vi "FillSurfaceRects.vi"(8 "No Error":errorcluster, 9 "Color":u32, 10 "Rects":T1[](array[typedef]), 11 "Dst [SDL_Surface *]":i64 format="%.0x") -> (0 "error out":errorcluster)   [LabVIEW 2026, in "SDL3.lvlib" / "Surface.lvlib"]
doc: "<B>Summary</B>\nPerform a fast fill of a set of rectangles with a specific color.\n\n<B>Remarks</B>\ncolor should be a pixel of the format used by the surface, and can be generated by SDL_MapRGB() or SDL_MapRGBA(). If the color value contains an alpha component then the destination is simply filled with that alpha information, no blending takes place.\n\nIf there is a clip rectangle set on the destination (set via SDL_SetSurfaceClipRect()), then this function will fill based on the intersection of the clip rectangle and rect."
uses:
  Surface.lvlib
  Rect/Rect--cluster.ctl
  <vilib>/Utility/error.llb/Error Cluster From Error Code.vi
  Error/Error.lvlib
  Lib/SDL3.dll
  Rect/Rect.lvlib
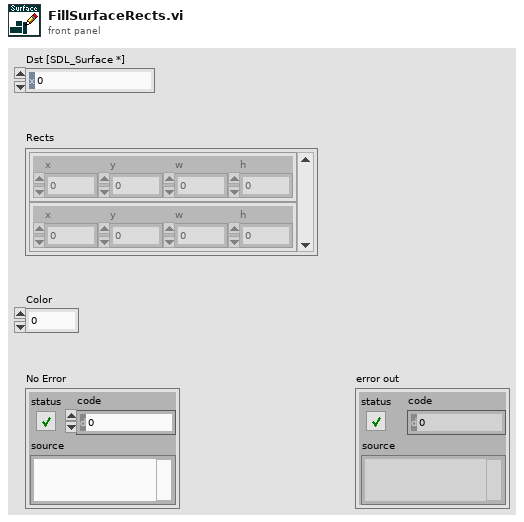
[diagram p1: front panel]
types:
  T1 = typedef "SDL3.lvlib/Rect.lvlib/Rect--cluster.ctl" = cluster{"x":i32, "y":i32, "w":i32, "h":i32}
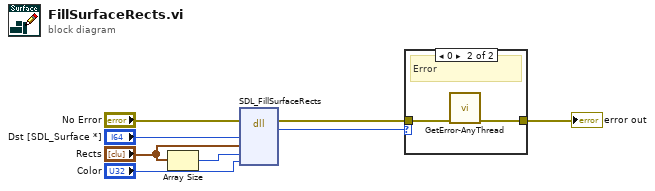
[diagram p0: block diagram]
diagram:
  n1 = Array Size(array="Rects") -> (size(s)=w1:i32)
  n2 = dll-call lib="C:/Users/saukko/Dev/LV-SDL3/Sources/SDL3/Lib/SDL3.*" fn="SDL_FillSurfaceRects"(error in="No Error", "dst"="Dst [SDL_Surface *]", "rects"="Rects", "count"=w1, "color"="Color") -> (error out=w3:errorcluster, "return type"=w2:i32)  [unwired: 6 in, 1 out]
  n3 = case shown="0" w2 {
    tunnel: w3 -> [w9 w11]
    tunnel: [w9 w10] -> w7
    frame Default {
      # "Ok"
    }
    frame 0 {
      # "Error"
      n4 = call "GetError-AnyThread.vi"("No Error"=w11) -> ("Error Out"=w10:errorcluster)  [unwired: 10 in]
    }
  }
  "error out" <- w7
